vi "Pressure Readout.vi"() -> ()   [LabVIEW 2018]
uses:
  <vilib>/DAQmx/read.llb/DAQmx Read (Analog DBL 1Chan 1Samp).vi
  <vilib>/DAQmx/create/channels.llb/DAQmx Create Channel (AI-Voltage-Basic).vi
  <vilib>/DAQmx/miscellaneous.llb/DAQmx Fill In Error Info.vi
panel:
  out "Pressure (in torr)":dbl
  in  "stop":bool
  out "Pressure Readout  (in Torr)":dbl(knob) scale=0.0..1000.0
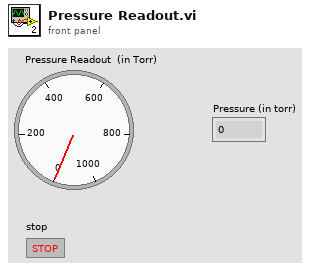
[diagram p1: front panel]
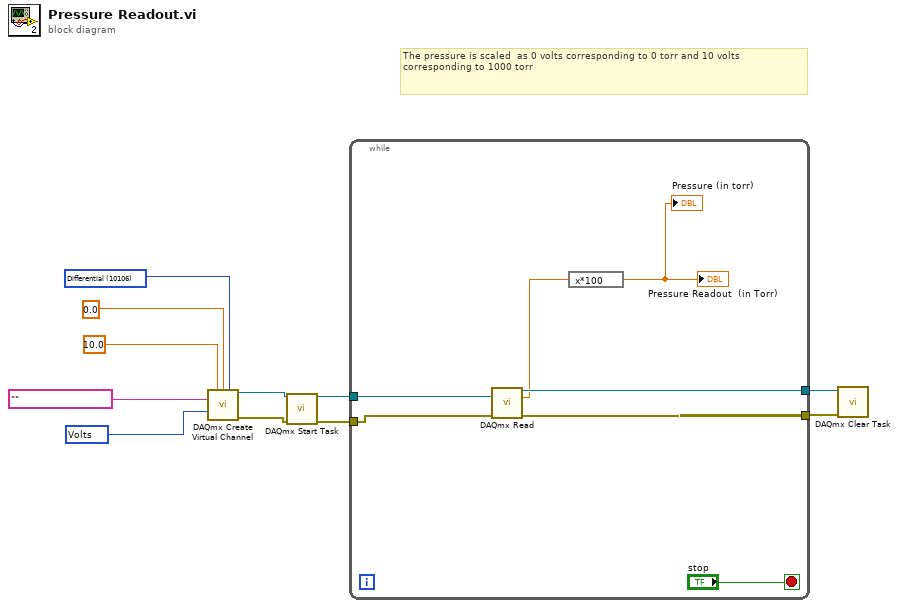
[diagram p0: block diagram]
diagram:
  w1 = 10348 items=["Volts"=10348, "From Custom Scale"=10065] ("units")
  w3 = 10106 items=["Default"=-1, "RSE"=10083, "NRSE"=10078, "Differential"=10106, "Pseudodifferential"=12529] ("input terminal configuration")
  # "The pressure is scaled  as 0 volts corresponding to 0 torr and 10 volts corresponding to 1000 torr"
  n1 = call-poly <vilib>:"DAQmx Create Virtual Channel.vi"("maximum value"=10.0, "minimum value"=0.0, "input terminal configuration"=w3, "physical channels"=tag "", "units"=w1) -> ("task out"=w11:refnum<k21>, "error out"=w10:errorcluster)  [unwired: 9 in]
  n2 = call <vilib>:"DAQmx Start Task.vi"("task/channels in"=w11, "error in"=w10) -> ("task out"=w9:refnum<k21>, "error out"=w7:errorcluster)  [unwired: 12 in]
  n3 = while {
    tunnel: w9 -> [w18]
    tunnel: [w17] -> w8
    tunnel: w7 -> [w16]
    tunnel: [w15] -> w6
    stop <- "stop" stop-if-true
    n4 = call-poly <vilib>:"DAQmx Read.vi"("task/channels in"=w18, "error in"=w16) -> ("task out"=w17:refnum<k21>, "data"=w14:dbl, "error out"=w15:errorcluster)  [unwired: 11 in]
    n5 = expression code="x*100"(w14) -> (→"Pressure Readout  (in Torr)" →"Pressure (in torr)":dbl)
  }
  n6 = call <vilib>:"DAQmx Clear Task.vi"("task in"=w8, "error in"=w6) -> ()  [unwired: 13 in, 1 out]
